vi "checkROIAndUpdate.vi"(5 "Settings.number of cam":dbl, 9 "Settings.CamSettings 3":T1={"Cam 0"={"position"=0.0, "pixelsize"=0.0, "start"=0.0, "end"=0.0, "center"=0.0, "Lens"=enum."FL1-f8x08", "Forward"=enum."off", "Spec_Calib_file 2"=path "Y:/100TWdata/ESMCalib/datFwd.txt", "map"=path "Y:/100TWdata/ESMCalib/mapFwd.txt", "y size"=0, "UserROI"={"Width"={"Value"=0.0, "Min"=0.0, "Max"=0.0, "StepSize"=0.0, "Tolerance"=0.0, "ValueActual"=0.0}, "Hight"={"Value"=0.0, "Min"=0.0, "Max"=0.0, "StepSize"=0.0, "Tolerance"=0.0, "ValueActual"=0.0}, "OffsetX"={"Value"=0.0, "Min"=0.0, "Max"=0.0, "StepSize"=0.0, "Tolerance"=0.0, "ValueActual"=0.0}, "OffsetY"={"Value"=0.0, "Min"=0.0, "Max"=0.0, "StepSize"=0.0, "Tolerance"=0.0, "ValueActual"=0.0}}, "CamMaxPixel"={"X"=0, "Y"=0}, "CamROI"={"Width"=0.0, "Hight"=0.0, "OffsetX"=0.0, "OffsetY"=0.0}}, "Cam 1"={"position"=0.0, "pixelsize"=0.0, "start"=0.0, "end"=0.0, "center"=0.0, "Lens"=enum."FL1-f8x08", "Forward"=enum."off", "Spec_Calib_file 2"=path "Y:/100TWdata/ESMCalib/datFwd.txt", "map"=path "Y:/100TWdata/ESMCalib/mapFwd.txt", "y size"=0, "UserROI"={"Width"={"Value"=0.0, "Min"=0.0, "Max"=0.0, "StepSize"=0.0, "Tolerance"=0.0, "ValueActual"=0.0}, "Hight"={"Value"=0.0, "Min"=0.0, "Max"=0.0, "StepSize"=0.0, "Tolerance"=0.0, "ValueActual"=0.0}, "OffsetX"={"Value"=0.0, "Min"=0.0, "Max"=0.0, "StepSize"=0.0, "Tolerance"=0.0, "ValueActual"=0.0}, "OffsetY"={"Value"=0.0, "Min"=0.0, "Max"=0.0, "StepSize"=0.0, "Tolerance"=0.0, "ValueActual"=0.0}}, "CamMaxPixel"={"X"=0, "Y"=0}, "CamROI"={"Width"=0.0, "Hight"=0.0, "OffsetX"=0.0, "OffsetY"=0.0}}, "Cam 2"={"position"=0.0, "pixelsize"=0.0, "start"=0.0, "end"=0.0, "center"=0.0, "Lens"=enum."FL1-f8x08", "Forward"=enum."off", "Spec_Calib_file 2"=path "Y:/100TWdata/ESMCalib/datFwd.txt", "map"=path "Y:/100TWdata/ESMCalib/mapFwd.txt", "y size"=0, "UserROI"={"Width"={"Value"=0.0, "Min"=0.0, "Max"=0.0, "StepSize"=0.0, "Tolerance"=0.0, "ValueActual"=0.0}, "Hight"={"Value"=0.0, "Min"=0.0, "Max"=0.0, "StepSize"=0.0, "Tolerance"=0.0, "ValueActual"=0.0}, "OffsetX"={"Value"=0.0, "Min"=0.0, "Max"=0.0, "StepSize"=0.0, "Tolerance"=0.0, "ValueActual"=0.0}, "OffsetY"={"Value"=0.0, "Min"=0.0, "Max"=0.0, "StepSize"=0.0, "Tolerance"=0.0, "ValueActual"=0.0}}, "CamMaxPixel"={"X"=0, "Y"=0}, "CamROI"={"Width"=0.0, "Hight"=0.0, "OffsetX"=0.0, "OffsetY"=0.0}}, "Cam 3"={"position"=0.0, "pixelsize"=0.0, "start"=0.0, "end"=0.0, "center"=0.0, "Lens"=enum."FL1-f8x08", "Forward"=enum."off", "Spec_Calib_file 2"=path "Y:/100TWdata/ESMCalib/datFwd.txt", "map"=path "Y:/100TWdata/ESMCalib/mapFwd.txt", "y size"=0, "UserROI"={"Width"={"Value"=0.0, "Min"=0.0, "Max"=0.0, "StepSize"=0.0, "Tolerance"=0.0, "ValueActual"=0.0}, "Hight"={"Value"=0.0, "Min"=0.0, "Max"=0.0, "StepSize"=0.0, "Tolerance"=0.0, "ValueActual"=0.0}, "OffsetX"={"Value"=0.0, "Min"=0.0, "Max"=0.0, "StepSize"=0.0, "Tolerance"=0.0, "ValueActual"=0.0}, "OffsetY"={"Value"=0.0, "Min"=0.0, "Max"=0.0, "StepSize"=0.0, "Tolerance"=0.0, "ValueActual"=0.0}}, "CamMaxPixel"={"X"=0, "Y"=0}, "CamROI"={"Width"=0.0, "Hight"=0.0, "OffsetX"=0.0, "OffsetY"=0.0}}}, 11 "ROI in":T8) -> (1 "Settings.CamSettings 2":T1={"Cam 0"={"position"=0.0, "pixelsize"=0.0, "start"=0.0, "end"=0.0, "center"=0.0, "Lens"=enum."FL1-f8x08", "Forward"=enum."off", "Spec_Calib_file 2"=path "Y:/100TWdata/ESMCalib/datFwd.txt", "map"=path "Y:/100TWdata/ESMCalib/mapFwd.txt", "y size"=0, "UserROI"={"Width"={"Value"=0.0, "Min"=0.0, "Max"=0.0, "StepSize"=0.0, "Tolerance"=0.0, "ValueActual"=0.0}, "Hight"={"Value"=0.0, "Min"=0.0, "Max"=0.0, "StepSize"=0.0, "Tolerance"=0.0, "ValueActual"=0.0}, "OffsetX"={"Value"=0.0, "Min"=0.0, "Max"=0.0, "StepSize"=0.0, "Tolerance"=0.0, "ValueActual"=0.0}, "OffsetY"={"Value"=0.0, "Min"=0.0, "Max"=0.0, "StepSize"=0.0, "Tolerance"=0.0, "ValueActual"=0.0}}, "CamMaxPixel"={"X"=0, "Y"=0}, "CamROI"={"Width"=0.0, "Hight"=0.0, "OffsetX"=0.0, "OffsetY"=0.0}}, "Cam 1"={"position"=0.0, "pixelsize"=0.0, "start"=0.0, "end"=0.0, "center"=0.0, "Lens"=enum."FL1-f8x08", "Forward"=enum."off", "Spec_Calib_file 2"=path "Y:/100TWdata/ESMCalib/datFwd.txt", "map"=path "Y:/100TWdata/ESMCalib/mapFwd.txt", "y size"=0, "UserROI"={"Width"={"Value"=0.0, "Min"=0.0, "Max"=0.0, "StepSize"=0.0, "Tolerance"=0.0, "ValueActual"=0.0}, "Hight"={"Value"=0.0, "Min"=0.0, "Max"=0.0, "StepSize"=0.0, "Tolerance"=0.0, "ValueActual"=0.0}, "OffsetX"={"Value"=0.0, "Min"=0.0, "Max"=0.0, "StepSize"=0.0, "Tolerance"=0.0, "ValueActual"=0.0}, "OffsetY"={"Value"=0.0, "Min"=0.0, "Max"=0.0, "StepSize"=0.0, "Tolerance"=0.0, "ValueActual"=0.0}}, "CamMaxPixel"={"X"=0, "Y"=0}, "CamROI"={"Width"=0.0, "Hight"=0.0, "OffsetX"=0.0, "OffsetY"=0.0}}, "Cam 2"={"position"=0.0, "pixelsize"=0.0, "start"=0.0, "end"=0.0, "center"=0.0, "Lens"=enum."FL1-f8x08", "Forward"=enum."off", "Spec_Calib_file 2"=path "Y:/100TWdata/ESMCalib/datFwd.txt", "map"=path "Y:/100TWdata/ESMCalib/mapFwd.txt", "y size"=0, "UserROI"={"Width"={"Value"=0.0, "Min"=0.0, "Max"=0.0, "StepSize"=0.0, "Tolerance"=0.0, "ValueActual"=0.0}, "Hight"={"Value"=0.0, "Min"=0.0, "Max"=0.0, "StepSize"=0.0, "Tolerance"=0.0, "ValueActual"=0.0}, "OffsetX"={"Value"=0.0, "Min"=0.0, "Max"=0.0, "StepSize"=0.0, "Tolerance"=0.0, "ValueActual"=0.0}, "OffsetY"={"Value"=0.0, "Min"=0.0, "Max"=0.0, "StepSize"=0.0, "Tolerance"=0.0, "ValueActual"=0.0}}, "CamMaxPixel"={"X"=0, "Y"=0}, "CamROI"={"Width"=0.0, "Hight"=0.0, "OffsetX"=0.0, "OffsetY"=0.0}}, "Cam 3"={"position"=0.0, "pixelsize"=0.0, "start"=0.0, "end"=0.0, "center"=0.0, "Lens"=enum."FL1-f8x08", "Forward"=enum."off", "Spec_Calib_file 2"=path "Y:/100TWdata/ESMCalib/datFwd.txt", "map"=path "Y:/100TWdata/ESMCalib/mapFwd.txt", "y size"=0, "UserROI"={"Width"={"Value"=0.0, "Min"=0.0, "Max"=0.0, "StepSize"=0.0, "Tolerance"=0.0, "ValueActual"=0.0}, "Hight"={"Value"=0.0, "Min"=0.0, "Max"=0.0, "StepSize"=0.0, "Tolerance"=0.0, "ValueActual"=0.0}, "OffsetX"={"Value"=0.0, "Min"=0.0, "Max"=0.0, "StepSize"=0.0, "Tolerance"=0.0, "ValueActual"=0.0}, "OffsetY"={"Value"=0.0, "Min"=0.0, "Max"=0.0, "StepSize"=0.0, "Tolerance"=0.0, "ValueActual"=0.0}}, "CamMaxPixel"={"X"=0, "Y"=0}, "CamROI"={"Width"=0.0, "Hight"=0.0, "OffsetX"=0.0, "OffsetY"=0.0}}}, 3 "new ROI":bool)   [LabVIEW 2013, in "MagAnalysis_Online.lvclass"]
uses:
  MagAnalysis_Online.lvclass
  ROIStartfromCam_typdef.ctl
  classicROI_typDef.ctl
  CamSettings_Typdef.ctl
  CamSettingSUB_TypDEf.ctl
  CamAndObj_TypDEf.ctl
  shared/OnOffTypeDef.ctl
  userROI.ctl
  shared/numericVariable_TypeDef.ctl
  CamRoiTypDef.ctl
  BaseDriver/BaseDriver.lvclass
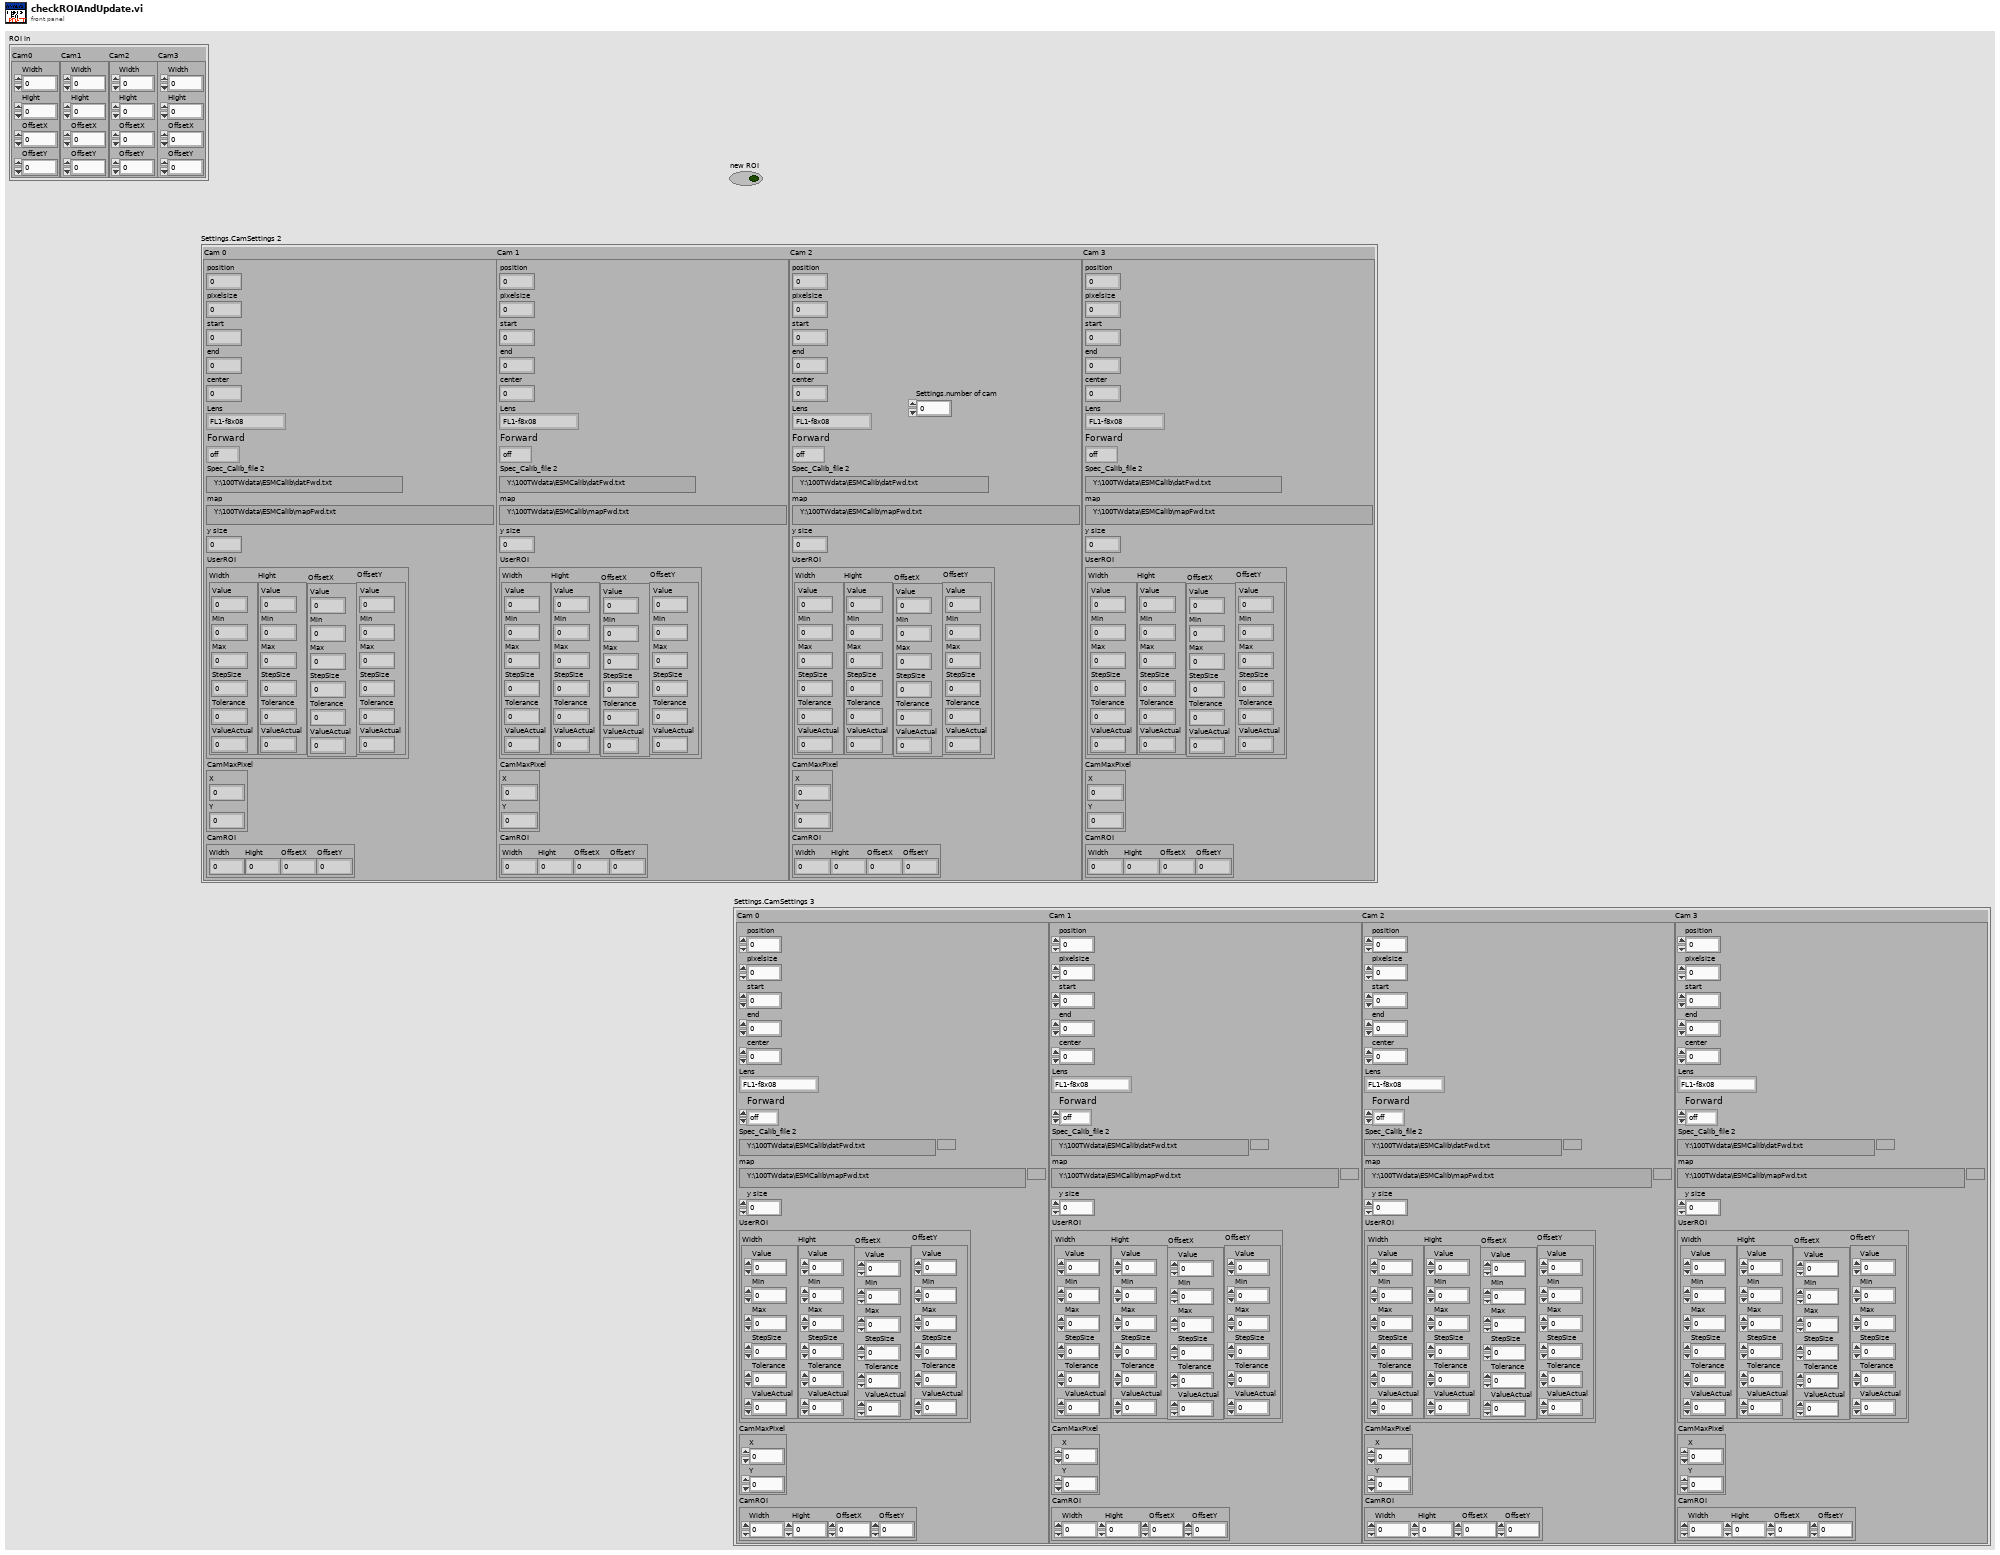
[diagram p1: front panel]
types:
  T1 = typedef "CamSettings_Typdef.ctl" = cluster{"Cam 0":T2, "Cam 1":T2, "Cam 2":T2, "Cam 3":T2}
  T2 = typedef "CamSettingSUB_TypDEf.ctl" = cluster{"position":dbl, "pixelsize":dbl, "start":dbl, "end":dbl, "center":dbl, "Lens":T3, "Forward":T4, "Spec_Calib_file 2":path, "map":path, "y size":i32, "UserROI":T5, "CamMaxPixel":cluster{"X":i32, "Y":i32}, "CamROI":T7}
  T3 = typedef "CamAndObj_TypDEf.ctl" = enum16{"FL1-f8x08", "FL1-f8x06", "FL1-f8", "ch300-f50", "FL2G-f8", "FL3M14-f8", "FL3M14-f8x08", "FL3M14-f8x08(2x2)"}
  T4 = typedef "OnOffTypeDef.ctl" = enum16{"off", "on"}
  T5 = typedef "userROI.ctl" = cluster{"Width":T6, "Hight":T6, "OffsetX":T6, "OffsetY":T6}
  T6 = typedef "BaseDriver.lvclass/numericVariable_TypeDef.ctl" = cluster{"Value":dbl, "Min":dbl, "Max":dbl, "StepSize":dbl, "Tolerance":dbl, "ValueActual":dbl}
  T7 = typedef "CamRoiTypDef.ctl" = cluster{"Width":dbl, "Hight":dbl, "OffsetX":dbl, "OffsetY":dbl}
  T8 = typedef "ROIStartfromCam_typdef.ctl" = cluster{"Cam0":T9, "Cam1":T9, "Cam2":T9, "Cam3":T9}
  T9 = typedef "classicROI_typDef.ctl" = cluster{"Width":dbl, "Hight":dbl, "OffsetX":dbl, "OffsetY":dbl}
  T10 = cluster{"Width":bool, "Hight":bool, "OffsetX":bool, "OffsetY":bool}
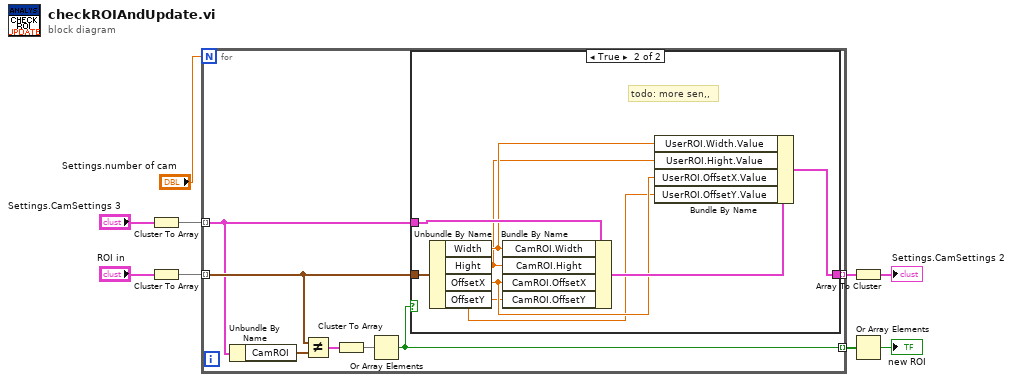
[diagram p0: block diagram]
diagram:
  n1 = Cluster To Array(cluster="Settings.CamSettings 3") -> (array=w7:T2[])
  n2 = Cluster To Array(cluster="ROI in") -> (array=w9:T9[])
  n3 = for {
    N: "Settings.number of cam" -> [_]
    tunnel: w9 -> [w14] mode=indexing
    tunnel: w7 -> [w11] mode=indexing
    tunnel: [w13] -> w3 mode=indexing
    tunnel: [w12] -> w1 mode=indexing
    n4 = Unbundle By Name(w11) -> ("CamROI"=w10:T7)
    n5 = Not Equal?(x=w14, y=w10) -> (x != y?=w16:T10)
    n6 = Cluster To Array(cluster=w16) -> (array=w15:bool[])
    n7 = Or Array Elements(Boolean array=w15) -> (logical OR=w13:bool)
    n8 = case shown="True" w13 {
      tunnel: w14 -> [_ w25]
      tunnel: w11 -> [w17 w24]
      tunnel: [w17 w18] -> w12
      frame False {
      }
      frame True {
        # "todo: more sen,,"
        n9 = Unbundle By Name(w25) -> ("Width"=w22:dbl, "Hight"=w21:dbl, "OffsetX"=w20:dbl, "OffsetY"=w19:dbl)
        n10 = Bundle By Name(cluster=w24, "CamROI.Width"=w22, "CamROI.Hight"=w21, "CamROI.OffsetX"=w20, "CamROI.OffsetY"=w19) -> (w23:T2)
        n11 = Bundle By Name(cluster=w23, "UserROI.Width.Value"=w22, "UserROI.Hight.Value"=w21, "UserROI.OffsetX.Value"=w20, "UserROI.OffsetY.Value"=w19) -> (w18:T2)
      }
    }
  }
  n12 = Array To Cluster(array=w1) -> (cluster=→"Settings.CamSettings 2":cluster{"[0]":T2, "[1]":T2, "[2]":T2, "[3]":T2})
  n13 = Or Array Elements(Boolean array=w3) -> (logical OR=→"new ROI":bool)
